vi "Init UI.vi"(8 "error in (no error)":errorcluster, 11 "Effect Unit in":refnum<class "Effect Unit.lvclass">) -> (0 "error out":errorcluster, 3 "Effect Unit out":refnum<class "Effect Unit.lvclass">)   [LabVIEW 2019, in "Effect Unit.lvclass"]
uses:
  Effect Unit.lvclass
  Libraries/Messaging/Messaging.lvlib
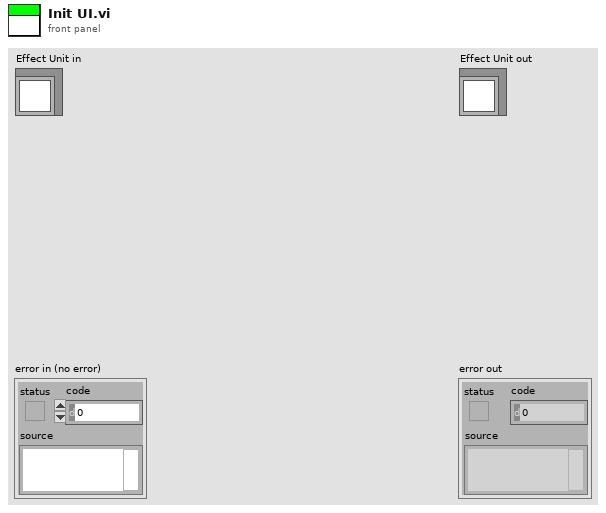
[diagram p1: front panel]
types:
  T1 = typedef "Effect Unit.lvclass/Effect Info.ctl" = cluster{"ID":string, "Message Queue":refnum<queue>, "Effect Interface":refnum<class "Effect Interface.lvclass">}
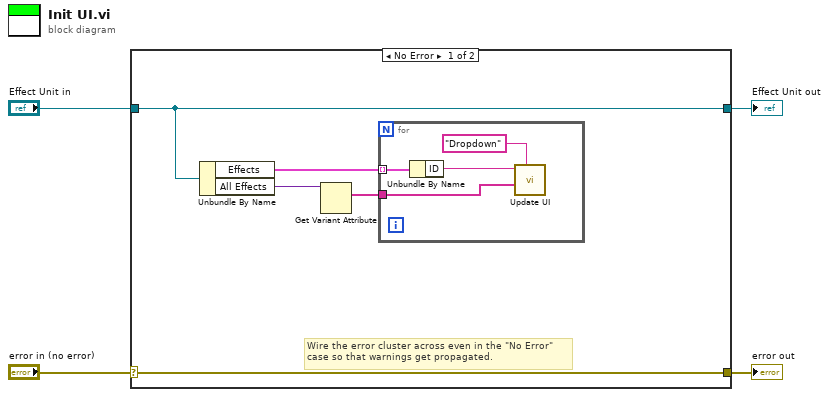
[diagram p0: block diagram]
diagram:
  n1 = case shown="No Error" "error in (no error)" {
    selector: "error in (no error)" -> [w9 w15]
    tunnel: [w9 w15] -> w3
    tunnel: [w8 w14] -> w1
    tunnel: "Effect Unit in" -> [w8 w14]
    frame No Error {
      # "Wire the error cluster across even in the \"No Error\"\ncase so that warnings get propagated."
      n2 = Unbundle By Name(w8) -> ("Effects"=w5:T1[], "All Effects"=w7:variant)
      n3 = Get Variant Attribute(Variant=w7) -> (names=w6:string[])  [unwired: 3 in, 3 out]
      n4 = for {
        tunnel: w5 -> [w13] mode=indexing
        tunnel: w6 -> [w10]
        n5 = Unbundle By Name(w13) -> ("ID"=w11:string)
        n6 = call "Update UI.vi"("Message (Value Change)"="Dropdown", "Data"=w10, "ID"=w11) -> ()  [unwired: 8 in, 1 out]
      }
    }
    frame Error {
    }
  }
  "error out" <- w3
  "Effect Unit out" <- w1
